vi "Add Library To Project.vi"(8 "error in":errorcluster, 11 "Script Strategy in":refnum<class "Script Strategy.lvclass">) -> (0 "error out":errorcluster)   [LabVIEW 2021, in "_Create From Template.lvlib" / "Script Strategy.lvlib" / "Script Strategy.lvclass"]
uses:
  Script Strategy.lvclass
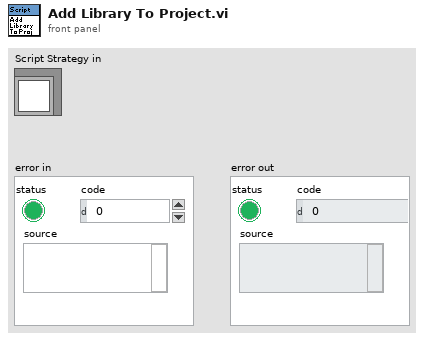
[diagram p1: front panel]
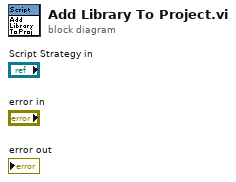
[diagram p0: block diagram]
diagram:
